vi "time_folder.vi"(11 "base path":path) -> (0 "error out":errorcluster, 3 "folder path":path)   [LabVIEW 2016]
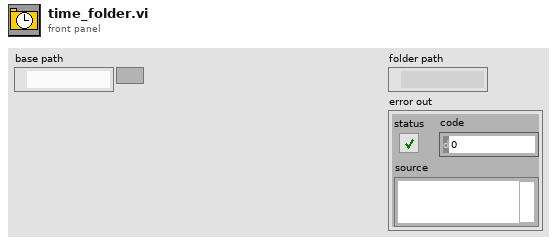
[diagram p1: front panel]
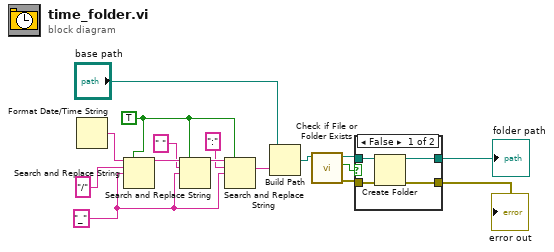
[diagram p0: block diagram]
diagram:
  w4 = TRUE ("replace all? (F)")
  w7 = "_" ("replace string (\"\")")
  n1 = Format Date/Time String() -> (date/time string=w12:string)  [unwired: 3 in]
  n2 = Search and Replace String(replace all?=w4, input string=w12, search string="/", replace string=w7) -> (result string=w10:string)  [unwired: 4 in, 3 out]
  n3 = Search and Replace String(replace all?=w4, input string=w10, search string=" ", replace string=w7) -> (result string=w8:string)  [unwired: 4 in, 3 out]
  n4 = Search and Replace String(replace all?=w4, input string=w8, search string=":", replace string=w7) -> (result string=w5:string)  [unwired: 4 in, 3 out]
  n5 = Build Path(base path="base path", name or relative path=w5) -> (appended path=w13:path)
  n6 = call <vilib>:"Check if File or Folder Exists.vi"("path"=w13) -> ("error out"=w16:errorcluster, "file or folder exists?"=w14:bool, "dup path"=w15:path)  [unwired: 8 in]
  n7 = case shown="False" w14 {
    tunnel: w15 -> [w20 w22]
    tunnel: w16 -> [w19 w21]
    tunnel: [w18 w22] -> w2
    tunnel: [w17 w21] -> w1
    frame False {
      n8 = Create Folder(path (use dialog)=w20, error in=w19) -> (created path=w18:path, error out=w17:errorcluster)  [unwired: 1 in, 1 out]
    }
    frame True {
    }
  }
  "folder path" <- w2
  "error out" <- w1
